vi "Name.vi"(8 "error in (no error)":errorcluster, 11 "Group in":refnum<class "Group.lvclass">) -> (0 "error out":errorcluster, 2 "Name":string, 3 "Group out":refnum<class "Group.lvclass">)   [LabVIEW 2020, in "VolatusConfig.lvlib" / "Group.lvclass"]
uses:
  Group.lvclass
  Group.lvclass/Group.ctl
  lv-cdm/CDM-Config/Config Element/Config Element.lvclass
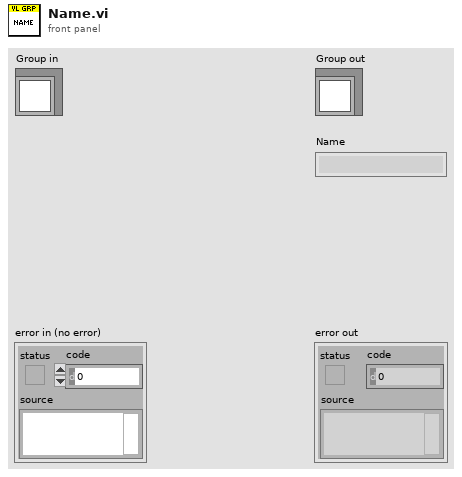
[diagram p1: front panel]
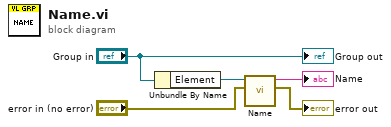
[diagram p0: block diagram]
diagram:
  n1 = Unbundle By Name("Group in") -> ("Element"=w4:refnum<class "Config Element.lvclass">)
  n2 = call "Name.vi"("error in (no error)"="error in (no error)", "Config Element in"=w4) -> ("error out"=→"error out":errorcluster, "Name"=→"Name":string)  [unwired: 8 in]
  "Group out" <- "Group in"
